vi "test mod cfg noops.vi"() -> ()   [LabVIEW 2013, in "TBM Tests.lvlib"]
uses:
  TBM Tests.lvlib
  module configuration/TBM module configuration.lvclass
  channel/TBM channel.lvclass
panel:
  out "warn 538305":errorcluster
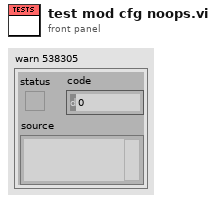
[diagram p1: front panel]
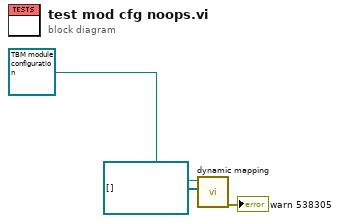
[diagram p0: block diagram]
diagram:
  n1 = call-dynamic "dynamic mapping.vi"("channels available"=refnum<class "TBM channel.lvclass">[] [], "module configuration in"=refnum<class "TBM module configuration.lvclass"> refnum ("module configuration")) -> ("error out"=→"warn 538305":errorcluster)  [unwired: 7 in, 2 out]
